vi "Actor Core.vi"(8 "error in":errorcluster, 11 "DAQ_Module in":refnum<class "DAQ_Module.lvclass">) -> (0 "error out":errorcluster, 3 "Actor out":refnum<class "Actor.lvclass">)   [LabVIEW 2025, in "DAQ_Module.lvlib" / "DAQ_Module.lvclass"]
doc: "<p>(<strong>Filename</strong>: <span class=\"dnl\">Actor Framework.lvlib:Actor.lvclass:Actor Core.vi</span>)</p>\n<p>Receives messages to the actor, reacts to them, and initiates any error handling that may shut the actor down.</p>\n<p>Descendant classes may override this VI to append parallel tasks for the actor to complete while it handles messages. Overrides use the <a href=\"nihelplauncher://docs/csh?context=lvcore_glang_udclass\">Call Parent Class Method</a> node.</p>"
uses:
  DAQ_Module.lvclass
  <vilib>/ActorFramework/Actor/Actor.lvclass
  DAQ_Module.lvclass/DAQ_Module.ctl
  <vilib>/ActorFramework/Actor/Actor.lvclass/Actor.ctl
  <vilib>/ActorFramework/Message Enqueuer/Message Enqueuer.lvclass/Message Enqueuer.ctl
  DAQ_Module Messages/ShowTask Msg/ShowTask Msg.lvclass/ShowTask Msg.ctl
  DAQ_Module Messages/StartTask Msg/StartTask Msg.lvclass/StartTask Msg.ctl
  DAQ_Module Messages/StopTask Msg/StopTask Msg.lvclass/StopTask Msg.ctl
  DAQ_Module Messages/StartRecord Msg/StartRecord Msg.lvclass/StartRecord Msg.ctl
  DAQ_Module Messages/StopRecord Msg/StopRecord Msg.lvclass/StopRecord Msg.ctl
  DAQ_Module Messages/SaveToTDMS Msg/SaveToTDMS Msg.lvclass/SaveToTDMS Msg.ctl
  DAQ_Module Messages/ClearData Msg/ClearData Msg.lvclass/ClearData Msg.ctl
  <vilib>/addons/_JKI Toolkits/State Machine/_JKI_lib_State_Machine.llb/Select State(s)_err__jki_lib_state_machine.vi
  a33a1397-74b9-4847-a830-d032f3b74699.vi
  <vilib>/ActorFramework/Message Enqueuer/Init from Existing Queue.vi
  <vilib>/ActorFramework/Message Enqueuer/Enqueue.vi
  Module/Module/Module Messages/PanelClose Msg/PanelClose Msg.lvclass
  <vilib>/ActorFramework/Stop Msg/Stop Msg.lvclass
  Module/Module/Module Messages/UI_Initialize Msg/UI_Initialize Msg.lvclass
  DAQ_Module Messages/CreateTasks Msg/CreateTasks Msg.lvclass
  DAQ_Module Messages/DestroyTask Msg/DestroyTask Msg.lvclass
  DAQ_Module Messages/ShowTask Msg/ShowTask Msg.lvclass
  DAQ_Module Messages/StartTask Msg/StartTask Msg.lvclass
  DAQ_Module Messages/StopTask Msg/StopTask Msg.lvclass
  DAQ_Module Messages/StartRecord Msg/StartRecord Msg.lvclass
  DAQ_Module Messages/StopRecord Msg/StopRecord Msg.lvclass
  DAQ_Module Messages/SaveToTDMS Msg/SaveToTDMS Msg.lvclass
  DAQ_Module Messages/ClearData Msg/ClearData Msg.lvclass
  <vilib>/addons/_JKI Toolkits/State Machine/_JKI_lib_State_Machine.llb/Periodic Trigger__ogtk__JKI-SM__jki_lib_state_machine.vi
  <vilib>/ActorFramework/Message Priority Queue/Priority Enqueue.vi
  <vilib>/Utility/TDMS File Viewer/TDMS - File Viewer (NXG Style).vi
  <vilib>/ActorFramework/Message Enqueuer/Message Enqueuer.lvclass
  Module/Module/Module/Module.lvclass
  <vilib>/Utility/TDMS File Viewer/NI_TDMS File Viewer.lvlib
panel:
  in  "Listbox":i32[](listbox)
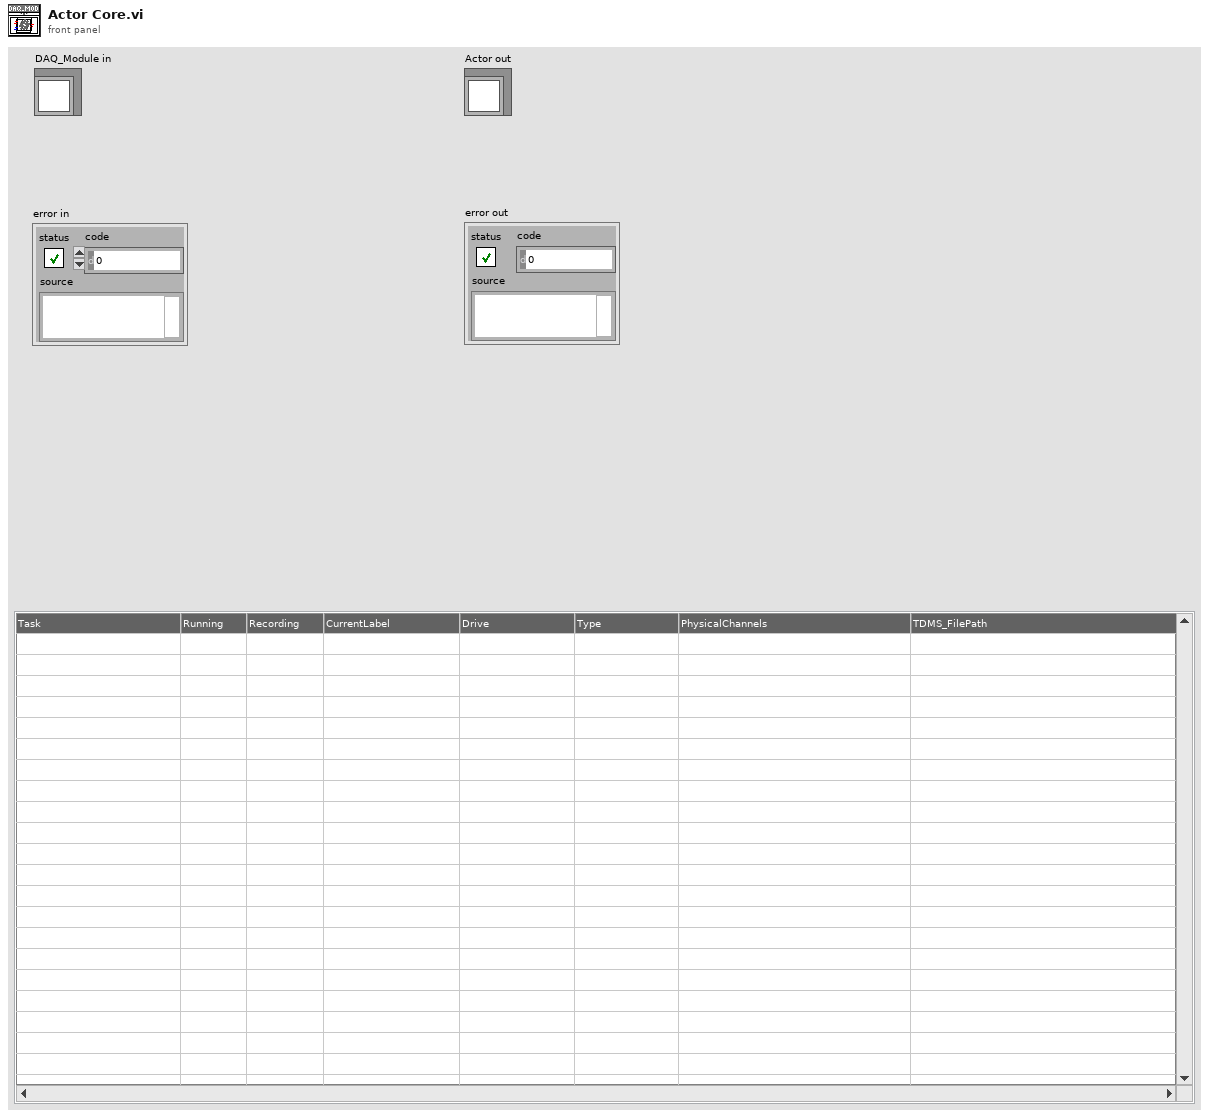
[diagram p1: front panel]
types:
  T1 = enum32{"Invalid", "Standard", "Closed", "Hidden", "Minimized", "Maximized"}
  T2 = enum32{"invalid app kind", "Development System", "Run Time System", "Student Edition", "Embedded LabVIEW", "Evaluation", "Custom"}
  T3 = typedef "Msg.ctl" = string
  T4 = cluster{"Core":cluster{"Current VI Reference":refnum<vi>, "Close Panel on Exit?":bool}, "Label":string[]}
  T5 = cluster{"Current VI Reference":refnum<vi>, "Close Panel on Exit?":bool}
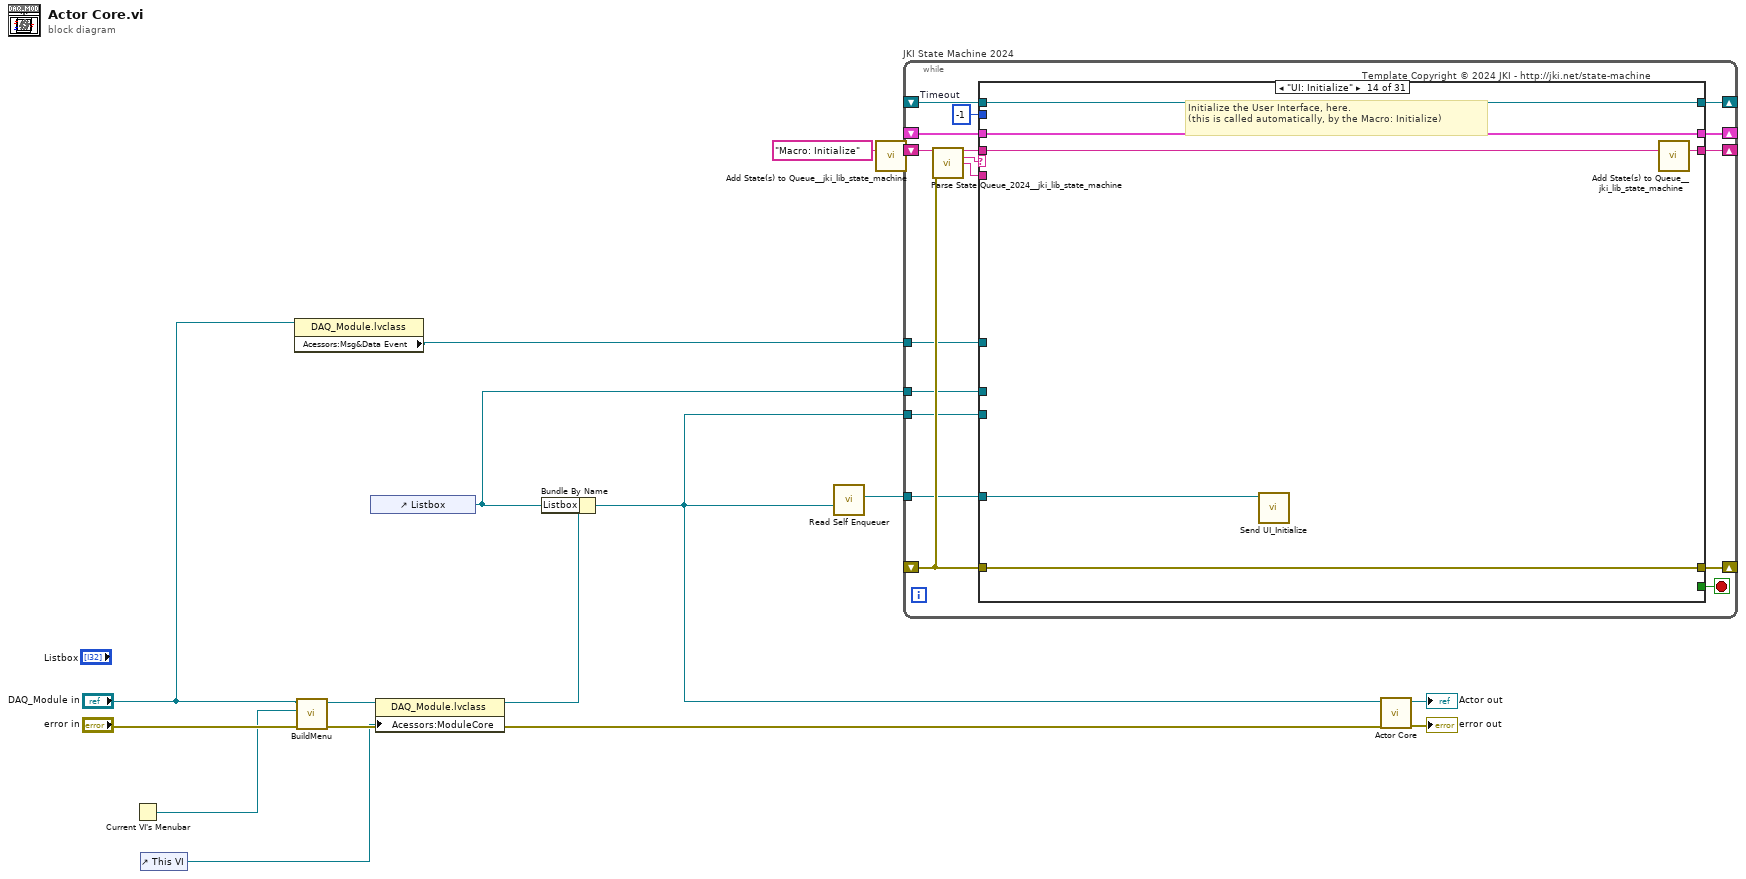
[diagram p0: block diagram]
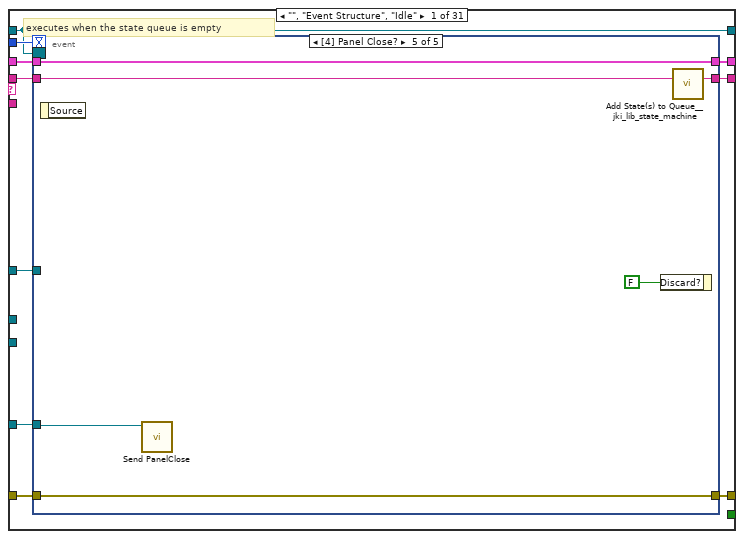
[diagram p2: hidden frame]
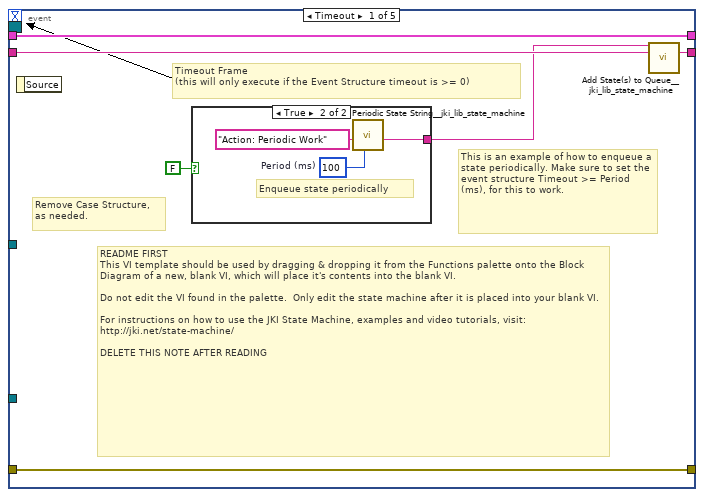
[diagram p3: hidden frame]
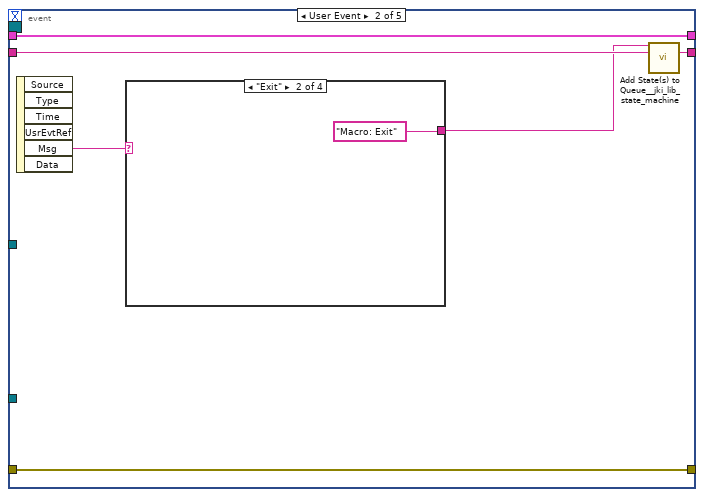
[diagram p5: hidden frame]
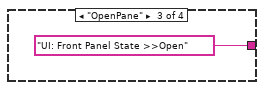
[diagram p7: hidden frame]
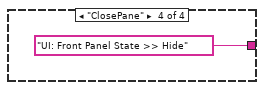
[diagram p8: hidden frame]
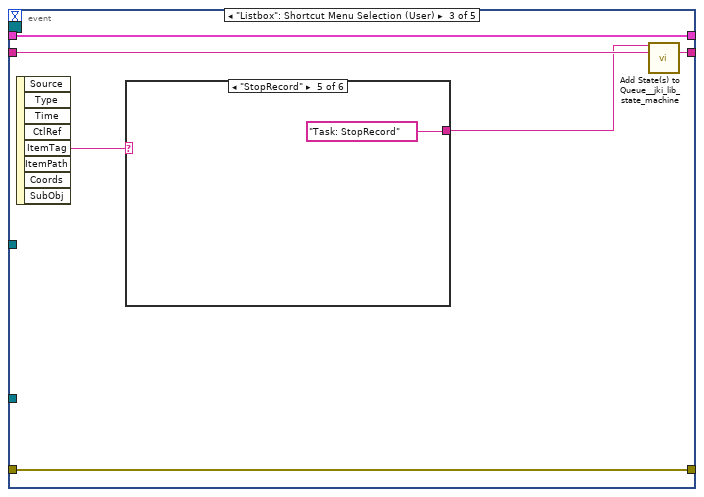
[diagram p9: hidden frame]
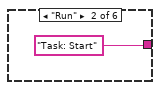
[diagram p11: hidden frame]
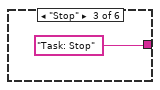
[diagram p12: hidden frame]
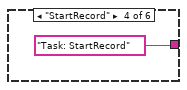
[diagram p13: hidden frame]
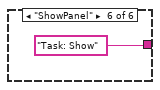
[diagram p14: hidden frame]
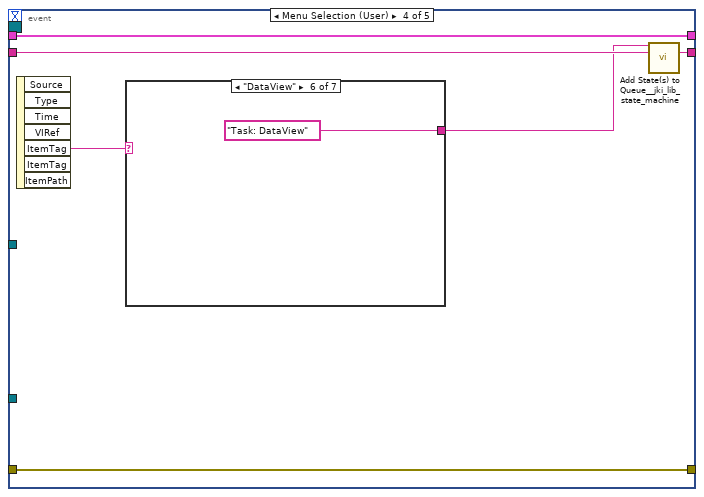
[diagram p15: hidden frame]
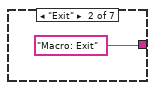
[diagram p17: hidden frame]
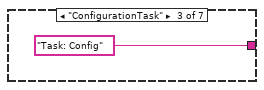
[diagram p18: hidden frame]
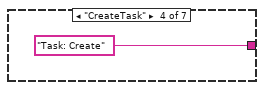
[diagram p19: hidden frame]
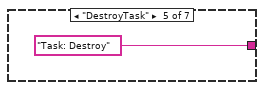
[diagram p20: hidden frame]
diagram:
  n1 = Current VI's Menubar() -> (w7:refnum<k9>)
  n2 = control-ref of="This VI"() -> (w1:refnum<vi>)
  n3 = property class="DAQ_Module.lvclass"(reference="DAQ_Module in") -> ("Acessors:Msg&Data Event"=w4:refnum<user-event>)  [unwired: 1 in, 2 out]
  n4 = call "BuildMenu.vi"("error in (no error)"="error in", "menu reference"=w7, "DAQ_Module in"="DAQ_Module in") -> ("error out"=w2:errorcluster, "DAQ_Module out"=w9:refnum<class "DAQ_Module.lvclass">)  [unwired: 7 in]
  n5 = control-ref of="Listbox"() -> (w6:refnum<vi>)
  n6 = property class="DAQ_Module.lvclass"(reference=w9, "Acessors:ModuleCore"=w1) -> (reference out=w3:refnum<class "DAQ_Module.lvclass">)  [unwired: 1 in, 1 out]
  n7 = Bundle By Name(cluster=w3, "Listbox"=w6) -> (w11:refnum<class "DAQ_Module.lvclass">)
  n8 = call <vilib>:"Read Self Enqueuer.vi"("Actor"=w11) -> ("Self Enqueuer"=w10:refnum<class "Message Enqueuer.lvclass">)  [unwired: 10 in]
  n9 = call <vilib>:"Add State(s) to Queue__jki_lib_state_machine.vi"("State(s) in (\"\")"="Macro: Initialize") -> ("States Out"=w13:string)  [unwired: 14 in]
  n10 = while "JKI State Machine 2024" {
    shift-right: [w25] -> _
    shift-left: _ -> [w24]
    shift-right: [w28] -> _
    shift-left: _ -> [w22]
    shift-right: [w27] -> _
    shift-left: w13 -> [w29]
    tunnel: w11 -> [w17]
    tunnel: w4 -> [w21]
    shift-right: [w20] -> _
    shift-left: _ -> [w19]
    tunnel: w10 -> [w18]
    tunnel: w6 -> [w16]
    stop <- w26 stop-if-true
    w23 = -1  # Timeout
    # "Template Copyright © 2024 JKI - http://jki.net/state-machine"
    n11 = call <vilib>:"Parse State Queue_2024__jki_lib_state_machine.vi"("State Queue"=w29, "Error In (no error)"=w22) -> ("Remaining States"=w31:string, "Current State"=w32:string, "Arguments"=w30:string)  [unwired: 11 in]
    n12 = case shown="\"UI: Initialize\"" w32 {
      selector: w32 -> [_ _ w96 _ _ _ _ _ _ _ _ _ _ _ _ _ _ _ _ _ _ _ _ _ _ _ _ _ _ _ _]
      tunnel: w31 -> [w42 w94 w100 w120 w131 w142 w147 w154 w161 w166 w173 w179 w184 w190 w195 w202 w214 w284 w290 w300 w305 w311 w317 w325 w335 w345 w357 w370 w388 w402 w411]
      tunnel: w30 -> [_ _ _ _ w126 _ _ _ _ _ _ _ _ _ _ w197 w208 _ _ _ _ _ _ _ _ _ _ _ _ _ _]
      tunnel: w24 -> [w40 w91 w98 w113 w128 w136 w144 _ w156 w163 w171 w177 w181 w188 w193 w200 w210 w281 w287 w298 w302 w306 w312 w322 w332 w342 w350 w367 w385 w399 w408]
      tunnel: [w39 w92 w102 w117 errorcluster {"status"=FALSE, "code"=0, "source"=""} ("error out") w140 w145 w151 w157 w164 w169 w174 w182 w187 w192 w198 w211 w282 w288 w295 w303 w309 w315 w323 w333 w343 w355 w368 w386 w400 w409] -> w28
      tunnel: w22 -> [w36 w92 w101 w117 w127 w140 w145 w151 w158 w164 w168 w175 w182 w187 w192 w199 w212 w282 w288 w295 w303 w309 w315 w323 w333 w343 w355 w368 w386 w400 w409]
      tunnel: [w41 w93 w99 w119 w130 w141 w146 w153 w160 w165 w172 w178 w183 w189 w194 w201 w213 w283 w289 w299 w304 w310 w316 w324 w334 w344 w356 w369 w387 w401 w410] -> w27
      tunnel: [_ _ _ _ _ TRUE _ _ _ _ _ _ _ _ _ _ _ _ _ _ _ _ _ _ _ _ _ _ _ _ _] -> w26
      tunnel: [w38 w91 w98 w118 w128 w136 w144 w152 w156 w163 w171 w177 w181 w188 w193 w200 w210 w281 w287 w298 w302 w306 w312 w322 w332 w342 w348 w367 w385 w399 w408] -> w25
      tunnel: w23 -> [w37 _ _ _ _ _ _ _ _ _ _ _ _ _ _ _ _ _ _ _ _ _ _ _ _ _ _ _ _ _ _]
      tunnel: w21 -> [w35 _ _ _ _ _ _ _ _ _ w167 _ _ _ _ _ _ _ _ _ _ _ _ _ _ _ _ _ _ _ _]
      tunnel: [w34 w90 w95 w107 w121 w138 w143 w149 w155 w162 w170 w176 w180 w186 w191 w196 w207 w280 w285 w291 w301 w308 w314 w321 w331 w341 w354 w366 w384 w398 w407] -> w20
      tunnel: w19 -> [w34 w90 w95 w107 w121 w138 w143 w149 w155 w162 _ w176 w180 w186 w191 w196 w207 w280 w285 w291 w301 w308 w314 w321 w331 w341 w354 w366 w384 w398 w407]
      tunnel: w18 -> [w33 _ _ _ _ w137 _ _ _ _ _ _ _ w185 _ _ _ _ _ _ _ w307 w313 w320 w330 w338 w353 w365 w382 _ _]
      tunnel: w17 -> [_ _ _ _ _ _ _ _ _ _ _ _ _ _ _ _ _ _ _ _ _ _ _ _ _ _ _ _ _ _ w406]
      tunnel: w16 -> [_ _ _ _ _ _ _ _ _ _ _ _ _ _ _ _ _ _ _ _ _ _ _ w319 w329 w339 w352 w364 w383 w397 _]
      frame "", "Event Structure", "Idle" {
        # "executes when the state queue is empty"
        n13 = event shown="[4] Panel Close?" {
          selector: w34 -> [_ _ _ _ _]
          dyn-events: _ -> [_ _ _ _ _]
          timeout: w37 -> [_ _ _ _ _]
          tunnel: w42 -> [w48 w57 w66 w77 w89]
          tunnel: [w47 w56 w65 w76 w88] -> w41
          tunnel: w40 -> [w45 w54 w63 w74 w86]
          tunnel: [w46 w55 w64 w75 w87] -> w39
          tunnel: w36 -> [w46 w55 w64 w75 w87]
          tunnel: [w45 w54 w63 w74 w86] -> w38
          tunnel: w35 -> [_ _ _ _ _]
          tunnel: w33 -> [_ _ _ _ w84]
          event Timeout {
            # "Remove Case Structure, as needed."
            # "This is an example of how to enqueue a state periodically. Make sure to set the event structure Timeout >= Period (ms), for this to work."
            # "README FIRST\nThis VI template should be used by dragging & dropping it from the Functions palette onto the Block Diagram of a new, blank VI, which will place it's contents into the blank VI.\n\nDo not edit the VI found in the palette.  Only edit the state machine after it is placed into your blank VI.\n\nFor instructions on how to use the JKI State Machine, examples and video tutorials, visit:\nhttp://jki.net/state-machine/\n\nDELETE THIS NOTE AFTER READING"
            # "Timeout Frame\n(this will only execute if the Event Structure timeout is >= 0)"
            n14 = event-data() -> ()  [unwired: 1 in, 1 out]
            n15 = case shown="True" FALSE {
              tunnel: [_ w51] -> w44
              frame False {
              }
              frame True {
                w49 = u32 100  # Period (ms)
                # "Enqueue state periodically"
                n16 = call <vilib>:"Periodic State String__jki_lib_state_machine.vi"("Period (ms)"=w49, "State"="Action: Periodic Work") -> ("State Out"=w51:string)  [unwired: 9 in]
              }
            }
            n17 = call <vilib>:"Add State(s) to Queue__jki_lib_state_machine.vi"("State(s) in Front (\"\")"=w44, "State(s) in (\"\")"=w48) -> ("States Out"=w47:string)  [unwired: 13 in]
          }
          event User Event {
            n18 = event-data() -> ("Msg"=w53:T3)  [unwired: 1 in, 5 out]
            n19 = case shown="\"Exit\"" w53 {
              tunnel: [_ "Macro: Exit" "UI: Front Panel State >>Open" "UI: Front Panel State >> Hide"] -> w52
              frame Default {
              }
              frame "Exit" {
              }
              frame "OpenPane" {
              }
              frame "ClosePane" {
              }
            }
            n20 = call <vilib>:"Add State(s) to Queue__jki_lib_state_machine.vi"("State(s) in Front (\"\")"=w52, "State(s) in (\"\")"=w57) -> ("States Out"=w56:string)  [unwired: 13 in]
          }
          event "Listbox": Shortcut Menu Selection (User) {
            n21 = event-data() -> ("ItemTag"=w62:string)  [unwired: 1 in, 7 out]
            n22 = case shown="\"StopRecord\"" w62 {
              tunnel: [_ "Task: Start" "Task: Stop" "Task: StartRecord" "Task: StopRecord" "Task: Show"] -> w61
              frame Default {
              }
              frame "Run" {
              }
              frame "Stop" {
              }
              frame "StartRecord" {
              }
              frame "StopRecord" {
              }
              frame "ShowPanel" {
              }
            }
            n23 = call <vilib>:"Add State(s) to Queue__jki_lib_state_machine.vi"("State(s) in Front (\"\")"=w61, "State(s) in (\"\")"=w66) -> ("States Out"=w65:string)  [unwired: 13 in]
          }
          event Menu Selection (User) {
            n24 = event-data() -> ("ItemTag"=w73:string)  [unwired: 1 in, 6 out]
            n25 = case shown="\"DataView\"" w73 {
              tunnel: [_ "Macro: Exit" "Task: Config" "Task: Create" "Task: Destroy" "Task: DataView" "Task: ClearData"] -> w72
              frame Default {
              }
              frame "Exit" {
              }
              frame "ConfigurationTask" {
              }
              frame "CreateTask" {
              }
              frame "DestroyTask" {
              }
              frame "DataView" {
              }
              frame "ClearData" {
              }
            }
            n26 = call <vilib>:"Add State(s) to Queue__jki_lib_state_machine.vi"("State(s) in Front (\"\")"=w72, "State(s) in (\"\")"=w77) -> ("States Out"=w76:string)  [unwired: 13 in]
          }
          event Panel Close? {
            n27 = event-data() -> ()  [unwired: 1 in, 1 out]
            n28 = call "Send PanelClose.vi"("Message Enqueuer"=w84) -> ()  [unwired: 9 in, 2 out]
            n29 = event-data("Discard?"=FALSE) -> ()  [unwired: 1 in, 1 out]
            n30 = call <vilib>:"Add State(s) to Queue__jki_lib_state_machine.vi"("State(s) in (\"\")"=w89) -> ("States Out"=w88:string)  [unwired: 14 in]
          }
        }
      }
      frame "---------- Core ----------" {
        # "Do not put any code in this frame.\n(it is a separator no-op)"
        n31 = call <vilib>:"Add State(s) to Queue__jki_lib_state_machine.vi"("State(s) in (\"\")"=w94) -> ("States Out"=w93:string)  [unwired: 14 in]
      }
      frame Default {
        w105 = 42 items=["No error", "Argument error", "Memory is full", "Out of zone", "End of file", "File already open", "Generic file I/O error", "File not found", "File permission error", "Disk is full", "Duplicate path", "Too many files open", "System feature not enabled", "Resource file not found", "Cannot add resource", "Resource not found", "Image not found", "Image memory error", "Pen does not exist", "Config type invalid", "Config token not found", "Config parse error", "Config memory error", "Bad external code format", "Bad external code offset", "External code not present", "Null window", "Destroy window error", "Null menu", "Print aborted", "Bad print record", "Print driver error", "Windows error during printing", "Memory error during printing", "Print dialog error", "Generic print error", "Invalid device refnum", "Device not found", "Device parameter error", "Device unit error", "Cannot open device", "Device call aborted", "Generic error", "Cancelled by user", "Object ID too low", "Object ID too high", "Object not in heap", "Unknown heap", "Unknown object (invalid DefProc)", "Unknown object (DefProc not in table)", "Message out of range", "Invalid (null) method", "Unknown message", "Manager call not supported", "Bad address", "Network operation in progress", "Network operation timed out", "Connection is busy", "Network attribute not supported", "Network error", "Address in use", "System out of memory", "Connection aborted", "Connection refused", "Not connected", "Already connected", "Connection closed", "Initialization error (interapplication manager)", "Bad occurrence", "Wait on unbound occurrence handler", "Occurrence queue overflow", "Datalog type conflict", "Unused", "Unrecognized type (interapplication manager)", "Memory corrupt", "Failed to make temporary DLL", "Old CIN version", "Drag socket not found", "Failed to load drop-object", "Failed to register OLE object", "Failed to release OLE object", "Format specifier type mismatch", "Unknown format specifier", "Too few format specifiers", "Too many format specifiers", "Scan failed", "Newer CIN version", "Error converting to variant", "Runtime menu error", "Password tampered", "Variant attribute not found", "Incompatible variant data type", "Event data is not available", "Event Store is not present", "Occurrence is not found", "Event Queue is not created", "Event info is not available", "Refnum passed is NULL", "Error retrieving Class GUID", "Error retrieving CoClass GUID", "Error retrieving TypeLib GUID.", "Bad built application magic bytes.", "Specific driver is different from the specific driver associated with the Logical Name.", "There is no session opened to the class driver.", "Max Error", "MAX - Error with config objects", "MAX - Error loading configuration", "MAX - Group not supported"]
        # "Current State"
        # "Do not delete, rename, or modify this frame.\n(this is used to capture unhandled states and typos)"
        # "Handle mistyped state name (developer tool)"
        n32 = Format Into String(format string="Software Exception: Unhandled State \"%s\"." ("message"), error in=w101, w96) -> (resulting string=w104:string, error out=w103:errorcluster)  [unwired: 1 in]
        n33 = call <vilib>:"Error Cluster From Error Code.vi"("show call chain? (False)"=TRUE, "error in (no error)"=w103, "error message (\"\")"=w104, "error code (0)"=w105) -> ("error out"=w102:errorcluster)  [unwired: 5 in]
        n34 = call <vilib>:"Add State(s) to Queue__jki_lib_state_machine.vi"("State(s) in (\"\")"=w100) -> ("States Out"=w99:string)  [unwired: 14 in]
      }
      frame "Initialize Core Data" {
        # "Do not delete, rename, or modify this frame.\n(this is used to determine panel behavior on exit)"
        # "originally closed?"
        # "exe?"
        # "If panel starts closed or is an EXE, then close it when we exit"
        n35 = property class="VI"() -> ("FP.State"=w110:T1)  [unwired: 2 in, 2 out]
        n36 = property class="App"() -> ("App.Kind"=w116:T2)  [unwired: 2 in, 2 out]
        n37 = control-ref of="Current VI Reference"() -> (w111:refnum<vi>)
        n38 = Equal?(x=w110, y=T1."Closed" ("Front Panel Window:State")) -> (x = y?=w108:bool)
        n39 = Equal?(x=w116, y=T2."Run Time System" ("Application:Kind")) -> (x = y?=w114:bool)
        n40 = Or(x=w108, y=w114) -> (x .or. y?=w112:bool)
        n41 = Bundle By Name(cluster=w113, "Core.Current VI Reference"=w111, "Core.Close Panel on Exit?"=w112) -> (w118:T4)
        n42 = call <vilib>:"Add State(s) to Queue__jki_lib_state_machine.vi"("State(s) in (\"\")"=w120) -> ("States Out"=w119:string)  [unwired: 14 in]
      }
      frame "Error Handler" {
        # "When running as sourcecode, this function will add previous state data to the error message to aid the developer in troubleshoot errors.\nIf run as an executable, no additional information is added to the error message."
        # "This state receives both Errors and Warnings which is how the Status of this wire can be FALSE"
        # "Unhandled Error -- Display it"
        # "Handle any errors or warnings here.\nYou can also output any states to clean-up after errors or warnings occur"
        # "Clear error or warning"
        n43 = disable-structure shown="Default" {
          disable-tunnel: w127 -> [w134 w135]
          disable-tunnel: w126 -> [w133 _]
          disable-tunnel: [w132 w135] -> w125
          frame condition #0 (active) {
            n44 = call <vilib>:"Append Error Details__jki_lib_state_machine.vi"("error in (no error)"=w134, "Previous State and Argument(s)"=w133) -> ("error out"=w132:errorcluster)  [unwired: 9 in]
          }
          frame condition #1 {
          }
        }
        n45 = call <vilib>:"General Error Handler.vi"("error in (no error)"=w125) -> ()  [unwired: 10 in, 5 out]
        n46 = call-poly <vilib>:"Select State(s)__jki_lib_state_machine.vi"("State(s) if True (\"\")"="/* Post Error States", "Select"=w125, "State(s) if False (\"\")"="/* Post Warning States") -> ("States Out"=w123:string)  [unwired: 12 in]
        n47 = call <vilib>:"Add State(s) to Queue__jki_lib_state_machine.vi"("State(s) in Front (\"\")"=w123, "State(s) in (\"\")"=w131) -> ("States Out"=w130:string)  [unwired: 13 in]
      }
      frame "Exit" {
        # "Do not put any code in this frame.\n(No errors that occur here will be handled.)"
        n48 = call <vilib>:"Send Normal Stop.vi"("Message Enqueuer"=w137) -> ()  [unwired: 10 in, 1 out]
        n49 = call <vilib>:"Add State(s) to Queue__jki_lib_state_machine.vi"("State(s) in (\"\")"=w142) -> ("States Out"=w141:string)  [unwired: 14 in]
      }
      frame "---------- Data ----------" {
        # "Do not put any code in this frame.\n(It is a separator no-op. You can make a copy of this frame to create a new Data frame)"
        n50 = call <vilib>:"Add State(s) to Queue__jki_lib_state_machine.vi"("State(s) in (\"\")"=w147) -> ("States Out"=w146:string)  [unwired: 14 in]
      }
      frame "Data: Initialize" {
        w148 = string[] []  # Label
        w150 = T5 {"Current VI Reference"=refnum, "Close Panel on Exit?"=FALSE}  # Core
        # "do not delete - used by framework"
        # "Data names and types of shift register data are defined by this bundle."
        # "Initialize the shift-register data, here.\n(data names are defined by what you wire into the bundle function)"
        n51 = Bundle("Core"=w150, "Label"=w148) -> (w152:T4)  [unwired: 1 in]
        n52 = call <vilib>:"Add State(s) to Queue__jki_lib_state_machine.vi"("State(s) in (\"\")"=w154) -> ("States Out"=w153:string)  [unwired: 14 in]
      }
      frame "Data: Cleanup" {
        # "Cleanup any data and references, here.\n(this is called automatically, by the Macro: Exit)"
        n53 = Unbundle By Name(w156) -> ("Core.Current VI Reference"=w159:refnum<vi>)
        n54 = Close Reference(reference=w159, error in (no error)=w158) -> (error out=w157:errorcluster)
        n55 = call <vilib>:"Add State(s) to Queue__jki_lib_state_machine.vi"("State(s) in (\"\")"=w161) -> ("States Out"=w160:string)  [unwired: 14 in]
      }
      frame "---------- Events ----------" {
        # "Do not put any code in this frame.\n(It is a separator no-op. You can make a copy of this frame to create a new UI frame)"
        n56 = call <vilib>:"Add State(s) to Queue__jki_lib_state_machine.vi"("State(s) in (\"\")"=w166) -> ("States Out"=w165:string)  [unwired: 14 in]
      }
      frame "Events: Register" {
        # "Do not put any code in this frame.\n(It is a separator no-op. You can make a copy of this frame to create a new UI frame)"
        n57 = register-events(error in=w168, w167) -> (reference out=w170:refnum<event-registration>, error out=w169:errorcluster)  [unwired: 1 in]
        n58 = call <vilib>:"Add State(s) to Queue__jki_lib_state_machine.vi"("State(s) in (\"\")"=w173) -> ("States Out"=w172:string)  [unwired: 14 in]
      }
      frame "Events: Unregister" {
        # "Do not put any code in this frame.\n(It is a separator no-op. You can make a copy of this frame to create a new UI frame)"
        n59 = Unregister For Events(event registration refnum=w176, error in=w175) -> (error out=w174:errorcluster)
        n60 = call <vilib>:"Add State(s) to Queue__jki_lib_state_machine.vi"("State(s) in (\"\")"=w179) -> ("States Out"=w178:string)  [unwired: 14 in]
      }
      frame "---------- UI ----------" {
        # "Do not put any code in this frame.\n(It is a separator no-op. You can make a copy of this frame to create a new UI frame)"
        n61 = call <vilib>:"Add State(s) to Queue__jki_lib_state_machine.vi"("State(s) in (\"\")"=w184) -> ("States Out"=w183:string)  [unwired: 14 in]
      }
      frame "UI: Initialize" {
        # "Initialize the User Interface, here.\n(this is called automatically, by the Macro: Initialize)"
        n62 = call "Send UI_Initialize.vi"("Message Enqueuer"=w185) -> ()  [unwired: 9 in, 2 out]
        n63 = call <vilib>:"Add State(s) to Queue__jki_lib_state_machine.vi"("State(s) in (\"\")"=w190) -> ("States Out"=w189:string)  [unwired: 14 in]
      }
      frame "UI: Uninitialize" {
        # "Cleanup the User Interface, here.\n(this is called automatically, by the Macro: Exit)"
        n64 = call <vilib>:"Add State(s) to Queue__jki_lib_state_machine.vi"("State(s) in (\"\")"=w195) -> ("States Out"=w194:string)  [unwired: 14 in]
      }
      frame "UI: Cursor Set" {
        # "Argument"
        # "Set and Unset Cursor Busy.\n(Usage: \"UI: Cursor Set >> Busy|Idle\")"
        n65 = case shown="\"Idle\", Default" w197 {
          tunnel: w199 -> [w204 w206]
          tunnel: [w203 w205] -> w198
          frame "Idle", Default {
            n66 = call <vilib>:"Unset Busy.vi"("error in (no error)"=w204) -> ("error out"=w203:errorcluster)  [unwired: 10 in]
          }
          frame "Busy" {
            n67 = call <vilib>:"Set Busy.vi"("error in (no error)"=w206) -> ("error out"=w205:errorcluster)  [unwired: 9 in, 1 out]
          }
        }
        n68 = call <vilib>:"Add State(s) to Queue__jki_lib_state_machine.vi"("State(s) in (\"\")"=w202) -> ("States Out"=w201:string)  [unwired: 14 in]
      }
      frame "UI: Front Panel State" {
        # "Argument"
        # "Set Front Panel Open or Closed\n(Usage: \"UI: Front Panel State >> Open|Close\")"
        n69 = Unbundle By Name(w210) -> ("Core.Current VI Reference"=w209:refnum<vi>)
        n70 = case shown="\"Maximize\", \"Maximized\"" w208 {
          tunnel: w212 -> [w220 w235 w246 w259 w272]
          tunnel: [w222 w236 w248 w261 w274] -> w211
          tunnel: w209 -> [w221 w233 w247 w260 w273]
          frame "Open", "Standard", Default {
            w215 = T1."Standard" ("State")
            n71 = property class="VI"(reference=w221, error in=w220) -> (reference out=w218:refnum<vi>, error out=w219:errorcluster, "FP.State"=w217:T1)
            n72 = Not Equal?(x=w217, y=w215) -> (x != y?=w216:bool)
            n73 = case shown="True" w216 {
              tunnel: [w226 w228] -> w222
              tunnel: w219 -> [w225 w228]
              tunnel: w218 -> [w224 _]
              tunnel: w215 -> [w223 _]
              frame True {
                n74 = invoke class="VI" method="FP.Open"(reference=w224, error in=w225, "Activate"=TRUE, "State"=w223) -> (error out=w226:errorcluster)  [unwired: 1 in, 4 out]
              }
              frame False {
              }
            }
          }
          frame "Close", "Closed" {
            n75 = property class="VI"(reference=w233, error in=w235) -> (reference out=w232:refnum<vi>, error out=w234:errorcluster, "FP.State"=w230:T1)
            n76 = Not Equal?(x=w230, y=T1."Closed" ("Front Panel Window:State")) -> (x != y?=w229:bool)
            n77 = case shown="True" w229 {
              tunnel: [w237 w240] -> w236
              tunnel: w234 -> [w237 w239]
              tunnel: w232 -> [_ w238]
              frame False {
              }
              frame True {
                n78 = invoke class="VI" method="FP.Close"(reference=w238, error in=w239) -> (error out=w240:errorcluster)  [unwired: 1 in, 2 out]
              }
            }
          }
          frame "Hidden", "Hide" {
            w241 = T1."Hidden" ("State")
            n79 = property class="VI"(reference=w247, error in=w246) -> (reference out=w244:refnum<vi>, error out=w245:errorcluster, "FP.State"=w243:T1)
            n80 = Not Equal?(x=w243, y=w241) -> (x != y?=w242:bool)
            n81 = case shown="True" w242 {
              tunnel: [w252 w253] -> w248
              tunnel: w245 -> [w251 w253]
              tunnel: w244 -> [w250 _]
              tunnel: w241 -> [w249 _]
              frame True {
                n82 = invoke class="VI" method="FP.Open"(reference=w250, error in=w251, "State"=w249) -> (error out=w252:errorcluster)  [unwired: 2 in, 4 out]
              }
              frame False {
              }
            }
          }
          frame "Minimize", "Minimized" {
            w254 = T1."Minimized" ("State")
            n83 = property class="VI"(reference=w260, error in=w259) -> (reference out=w257:refnum<vi>, error out=w258:errorcluster, "FP.State"=w256:T1)
            n84 = Not Equal?(x=w256, y=w254) -> (x != y?=w255:bool)
            n85 = case shown="True" w255 {
              tunnel: [w265 w266] -> w261
              tunnel: w258 -> [w264 w266]
              tunnel: w257 -> [w263 _]
              tunnel: w254 -> [w262 _]
              frame True {
                n86 = invoke class="VI" method="FP.Open"(reference=w263, error in=w264, "State"=w262) -> (error out=w265:errorcluster)  [unwired: 2 in, 4 out]
              }
              frame False {
              }
            }
          }
          frame "Maximize", "Maximized" {
            w267 = T1."Maximized" ("State")
            n87 = property class="VI"(reference=w273, error in=w272) -> (reference out=w270:refnum<vi>, error out=w271:errorcluster, "FP.State"=w269:T1)
            n88 = Not Equal?(x=w269, y=w267) -> (x != y?=w268:bool)
            n89 = case shown="True" w268 {
              tunnel: [w278 w279] -> w274
              tunnel: w271 -> [w277 w279]
              tunnel: w270 -> [w276 _]
              tunnel: w267 -> [w275 _]
              frame True {
                n90 = invoke class="VI" method="FP.Open"(reference=w276, error in=w277, "State"=w275) -> (error out=w278:errorcluster)  [unwired: 2 in, 4 out]
              }
              frame False {
              }
            }
          }
        }
        n91 = call <vilib>:"Add State(s) to Queue__jki_lib_state_machine.vi"("State(s) in (\"\")"=w214) -> ("States Out"=w213:string)  [unwired: 14 in]
      }
      frame "---------- Macro ----------" {
        # "Do not put any code in this frame.\n(It is a separator no-op. You can make a copy of this frame to create a new Macro frame)"
        n92 = call <vilib>:"Add State(s) to Queue__jki_lib_state_machine.vi"("State(s) in (\"\")"=w284) -> ("States Out"=w283:string)  [unwired: 14 in]
      }
      frame "Macro: Initialize" {
        # "Initialization Macro\n(This is called once, when the VI starts)"
        n93 = call <vilib>:"Add State(s) to Queue__jki_lib_state_machine.vi"("State(s) in Front (\"\")"="Data: Initialize\nInitialize Core Data\nEvents: Register\nUI: Initialize\nUI: Front Panel State >> Hide", "State(s) in (\"\")"=w290) -> ("States Out"=w289:string)  [unwired: 13 in]
      }
      frame "Macro: Exit" {
        # "Exit Macro\n(This is called once, when the VI exits)"
        n94 = Unbundle By Name(w298) -> ("Core.Close Panel on Exit?"=w293:bool)
        n95 = call <vilib>:"Conditional State String__jki_lib_state_machine.vi"("Do State(s)?"=w293, "State"="UI: Front Panel State >> Close") -> ("State Out"=w292:string)  [unwired: 7 in]
        n96 = call <vilib>:"Add State(s) to Queue__jki_lib_state_machine.vi"("State(s) in (\"\")"=w292, "State(s) at Back (\"\")"="UI: Uninitialize\nData: Cleanup\nEvents: Unregister\nExit") -> ("States Out"=w296:string)  [unwired: 13 in]
        n97 = call <vilib>:"Add State(s) to Queue__jki_lib_state_machine.vi"("State(s) in Front (\"\")"=w296, "State(s) in (\"\")"=w300) -> ("States Out"=w299:string)  [unwired: 13 in]
      }
      frame "---------- Task ----------" {
        # "Template Separator\n(You can make a copy of, or modify, this frame)"
        n98 = call <vilib>:"Add State(s) to Queue__jki_lib_state_machine.vi"("State(s) in (\"\")"=w305) -> ("States Out"=w304:string)  [unwired: 14 in]
      }
      frame "Task: Create" {
        n99 = call "Send CreateTasks.vi"("Message Enqueuer"=w307) -> ()  [unwired: 9 in, 2 out]
        n100 = call <vilib>:"Add State(s) to Queue__jki_lib_state_machine.vi"("State(s) in (\"\")"=w311) -> ("States Out"=w310:string)  [unwired: 14 in]
      }
      frame "Task: Destroy" {
        # "Template Separator\n(You can make a copy of, or modify, this frame)"
        n101 = call "Send DestroyTask.vi"("Message Enqueuer"=w313) -> ()  [unwired: 9 in, 2 out]
        n102 = call <vilib>:"Add State(s) to Queue__jki_lib_state_machine.vi"("State(s) in (\"\")"=w317) -> ("States Out"=w316:string)  [unwired: 14 in]
      }
      frame "Task: Show" {
        # "Your code here.\n(You can make a copy of, or modify, this frame)"
        n103 = call "GetTaskFormList.vi"("Listbox"=w319) -> ("Tasks"=w318:string[])  [unwired: 6 in, 4 out]
        n104 = for {
          tunnel: w320 -> [w327]
          tunnel: w318 -> [w326] mode=indexing
          n105 = call "Send ShowTask.vi"("Task"=w326, "Message Enqueuer"=w327) -> ()  [unwired: 8 in, 2 out]
        }
        n106 = call <vilib>:"Add State(s) to Queue__jki_lib_state_machine.vi"("State(s) in (\"\")"=w325) -> ("States Out"=w324:string)  [unwired: 14 in]
      }
      frame "Task: Start" {
        # "Template Separator\n(You can make a copy of, or modify, this frame)"
        n107 = call "GetTaskFormList.vi"("Listbox"=w329) -> ("Tasks"=w328:string[])  [unwired: 6 in, 4 out]
        n108 = for {
          tunnel: w330 -> [w337]
          tunnel: w328 -> [w336] mode=indexing
          n109 = call "Send StartTask.vi"("Task"=w336, "Message Enqueuer"=w337) -> ()  [unwired: 8 in, 2 out]
        }
        n110 = call <vilib>:"Add State(s) to Queue__jki_lib_state_machine.vi"("State(s) in (\"\")"=w335) -> ("States Out"=w334:string)  [unwired: 14 in]
      }
      frame "Task: Stop" {
        # "Template Separator\n(You can make a copy of, or modify, this frame)"
        n111 = call "GetTaskFormList.vi"("Listbox"=w339) -> ("Tasks"=w340:string[])  [unwired: 6 in, 4 out]
        n112 = for {
          tunnel: w338 -> [w347]
          tunnel: w340 -> [w346] mode=indexing
          n113 = call "Send StopTask.vi"("Task"=w346, "Message Enqueuer"=w347) -> ()  [unwired: 8 in, 2 out]
        }
        n114 = call <vilib>:"Add State(s) to Queue__jki_lib_state_machine.vi"("State(s) in (\"\")"=w345) -> ("States Out"=w344:string)  [unwired: 14 in]
      }
      frame "Task: StartRecord" {
        # "Template Separator\n(You can make a copy of, or modify, this frame)"
        n115 = call "GetTaskFormList.vi"("Listbox"=w352) -> ("Time"=w349:string[], "Tasks"=w351:string[])  [unwired: 6 in, 3 out]
        n116 = for {
          tunnel: w353 -> [w360]
          tunnel: w351 -> [w359] mode=indexing
          tunnel: w349 -> [w358] mode=indexing
          n117 = call "Send StartRecord.vi"("Label"=w358, "Task"=w359, "Message Enqueuer"=w360) -> ()  [unwired: 7 in, 2 out]
        }
        n118 = Bundle By Name(cluster=w350, "Label"=w349) -> (w348:T4)
        n119 = call <vilib>:"Add State(s) to Queue__jki_lib_state_machine.vi"("State(s) in (\"\")"=w357) -> ("States Out"=w356:string)  [unwired: 14 in]
      }
      frame "Task: StopRecord" {
        # "Template Separator\n(You can make a copy of, or modify, this frame)"
        n120 = call "GetTaskFormList.vi"("Listbox"=w364) -> ("Label"=w362:string[], "Tasks"=w363:string[], "appended path"=w361:path)  [unwired: 6 in, 2 out]
        n121 = for {
          tunnel: w365 -> [w380]
          tunnel: w363 -> [w378] mode=indexing
          tunnel: w362 -> [w377] mode=indexing
          shift-right: [w373] -> _
          shift-left: _ -> [w372]
          tunnel: w361 -> [w371]
          n122 = call "Send StopRecord.vi"("error in (no error)"=w372, "Label"=w377, "Task"=w378, "Message Enqueuer"=w380) -> ("error out"=w376:errorcluster, "Message Enqueuer out"=w379:refnum<class "Message Enqueuer.lvclass">)  [unwired: 6 in]
          n123 = call "Stall Data Flow.vim"("value in"=w376, "milliseconds to wait"=u32 10) -> ("value out"=w375:errorcluster)  [unwired: 1 out]
          n124 = call "Send SaveToTDMS.vi"("TDMS File Path"=w371, "error in (no error)"=w375, "Label"=w377, "Task"=w378, "Message Enqueuer"=w379) -> ("error out"=w373:errorcluster)  [unwired: 5 in, 1 out]
        }
        n125 = call <vilib>:"Add State(s) to Queue__jki_lib_state_machine.vi"("State(s) in (\"\")"=w370) -> ("States Out"=w369:string)  [unwired: 14 in]
      }
      frame "Task: ClearData" {
        # "Template Separator\n(You can make a copy of, or modify, this frame)"
        n126 = call "GetTaskFormList.vi"("Listbox"=w383) -> ("Tasks"=w381:string[])  [unwired: 6 in, 4 out]
        n127 = for {
          tunnel: w382 -> [w390]
          tunnel: w381 -> [w389] mode=indexing
          n128 = call "Send ClearData.vi"("Task"=w389, "Message Enqueuer"=w390) -> ()  [unwired: 8 in, 2 out]
        }
        n129 = call <vilib>:"Add State(s) to Queue__jki_lib_state_machine.vi"("State(s) in (\"\")"=w388) -> ("States Out"=w387:string)  [unwired: 14 in]
      }
      frame "Task: DataView" {
        # "Template Separator\n(You can make a copy of, or modify, this frame)"
        n130 = call "GetTaskFormList.vi"("Listbox"=w397) -> ("path"=w391:path)  [unwired: 6 in, 4 out]
        n131 = vi-ref "NI_TDMS File Viewer.lvlib:TDMS - File Viewer (NXG Style).vi"() -> (w396:refnum<vi>)
        n132 = property class="VI"(reference=w396) -> ("Name"=w395:string)  [unwired: 1 in, 2 out]
        n133 = Open VI Reference(type specifier VI Refnum (for type only)=refnum<vi> refnum, vi path=w395, options=128) -> (vi reference=w392:refnum<vi>)  [unwired: 3 in, 1 out]
        n134 = call-by-ref "Start Asynchronous Call"(reference=w392, "file in"=w391) -> ()  [unwired: 10 in, 4 out]
        n135 = call <vilib>:"Add State(s) to Queue__jki_lib_state_machine.vi"("State(s) in (\"\")"=w402) -> ("States Out"=w401:string)  [unwired: 14 in]
      }
      frame "Task: Config" {
        # "Template Separator\n(You can make a copy of, or modify, this frame)"
        n136 = property class="DAQ_Module.lvclass"(reference=w406) -> (reference out=w404:refnum<class "DAQ_Module.lvclass">, "Acessors:ModuleName"=w403:string)  [unwired: 1 in, 1 out]
        n137 = Unbundle By Name(w404) -> ("TaskConfig"=w405:refnum<data-value>)
        n138 = call "Config.vi"("Model Name"=w403, "TaskConfig"=w405) -> ()  [unwired: 10 in]
        n139 = call <vilib>:"Add State(s) to Queue__jki_lib_state_machine.vi"("State(s) in (\"\")"=w411) -> ("States Out"=w410:string)  [unwired: 14 in]
      }
    }
  }
  n140 = call-parent "Actor Core.vi"("error in"=w2, "Actor in"=w11) -> ("error out"=→"error out":errorcluster, "Actor out"=→"Actor out":refnum<class "Actor.lvclass">)  [unwired: 8 in]
